vi "Spectrometer iHR320 Control Panel (No Objects).vi"(8 "error in (no error)":errorcluster) -> (0 "error out":errorcluster)   [LabVIEW 2012]
doc: "(Dynamic) A user-level application that simulates the physical front panel of the Instrument. Provide the user with buttons to manually control features of the instrument, and provide indicators of its current state."
panel:
  in  "Set Filter":bool
  out "Filter Index":i32(ring)=1 items=["Filter 1"=1, "Empty"=2, "Empty"=3, "Empty"=4, "Filter 2"=5, "Filter 3"=6]
  in  "Filter Index Set":i32(ring)=1 items=["Filter 1"=1, "Empty"=2, "Empty"=3, "Empty"=4, "Filter 2"=5, "Filter 3"=6]
  in  "Copy actual to set":bool
  in  "Populate fields with member data":bool
  out "Grating":u16(ring)=1 items=["1200"=1, "600"=2]
  in  "Set Grating":bool
  in  "stop":bool
  in  "Read to control":bool
  in  "Read":bool
  in  "Go To Wavelength":bool
  in  "Set Slit":bool
  in  "Grating set":u16(ring)=1 items=["1200"=1, "600"=2]
  out "Wavelength":dbl[unit]
  in  "Wavelength Set":dbl[unit]
  out "Exit Slit":dbl[unit]
  in  "Exit Slit Set":dbl[unit]
  out "Entrance Slit":dbl[unit]
  in  "Entrance  set":dbl[unit]
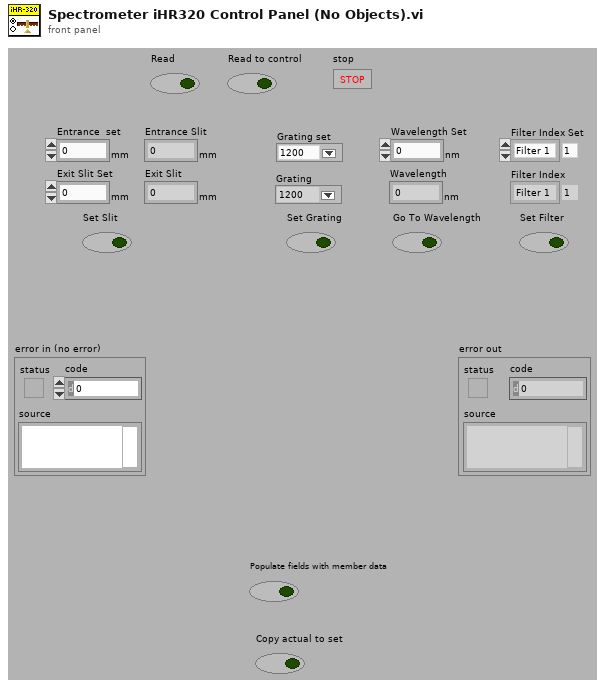
[diagram p1: front panel]
types:
  T1 = cluster{"Wavelength":dbl[unit], "Entrance slit width":dbl[unit], "Exit slit width":dbl[unit], "Init":cluster{"Initialized?":bool, "Emulating?":bool}, "Grating":cluster{"Groove Density":dbl[unit], "Blaze Wavelength":string, "Turrent Position":u16}, "RefNum":refnum<k7>, "Unique ID":string, "FW RefNum":refnum<k7>, "FW Unique ID":string, "Filter Index":i32}
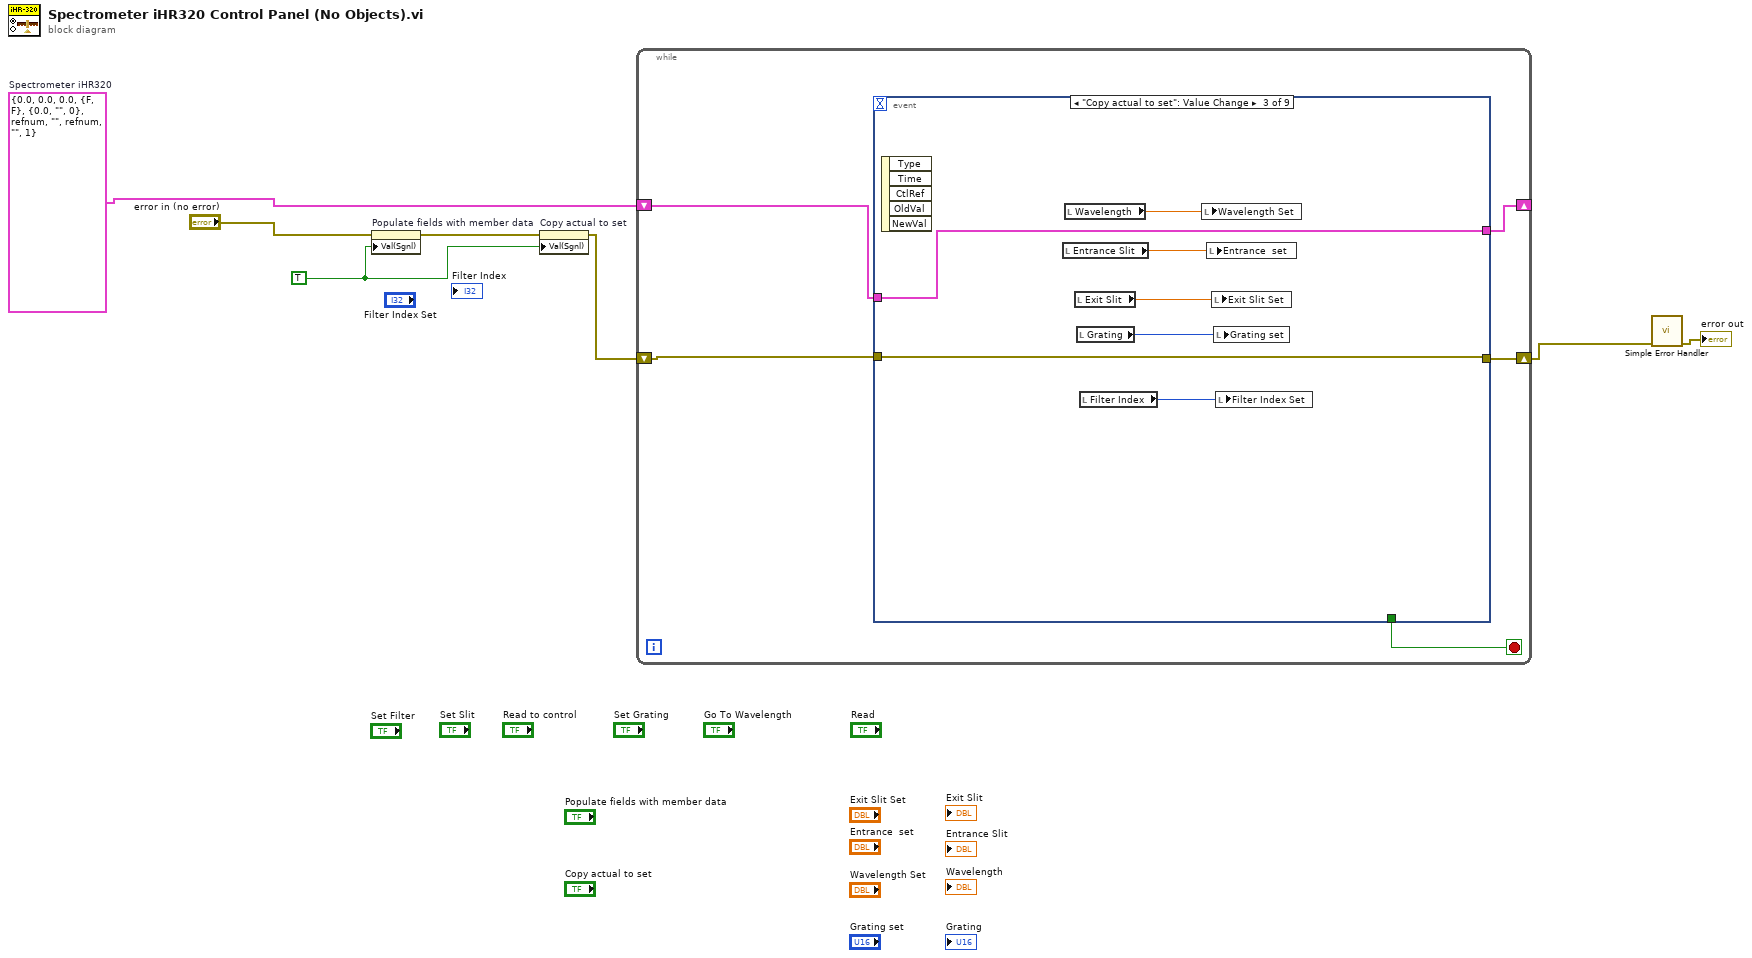
[diagram p0: block diagram]
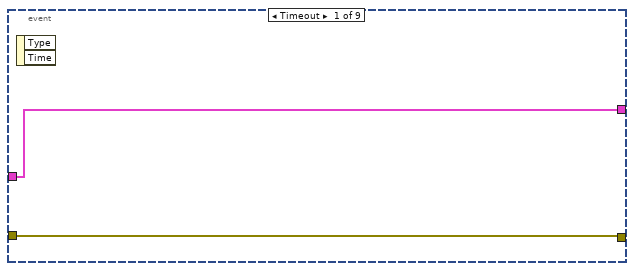
[diagram p2: hidden frame]
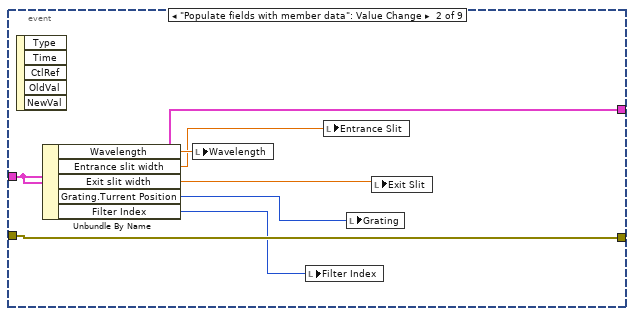
[diagram p3: hidden frame]
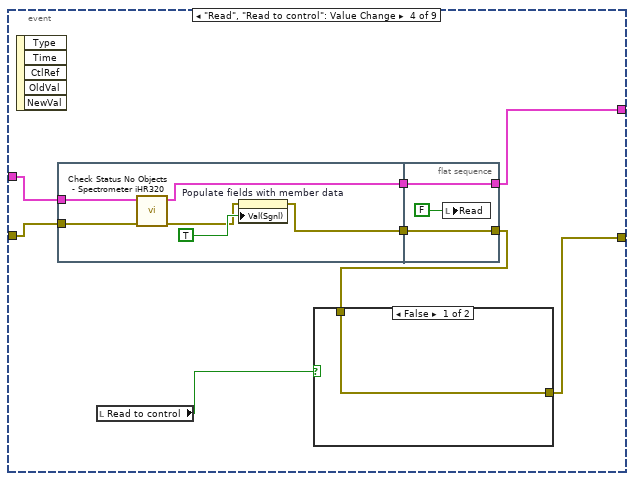
[diagram p4: hidden frame]
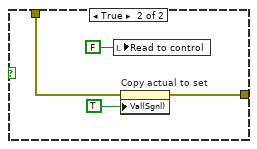
[diagram p5: hidden frame]
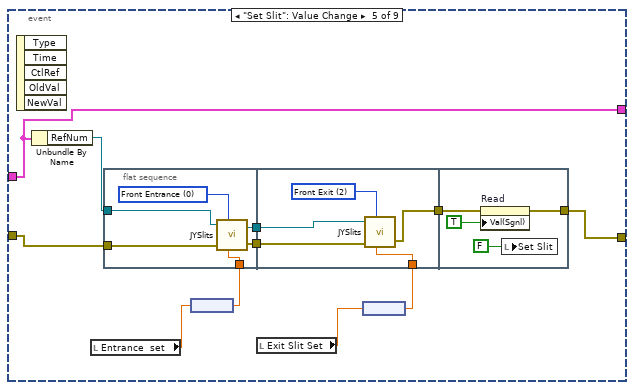
[diagram p6: hidden frame]
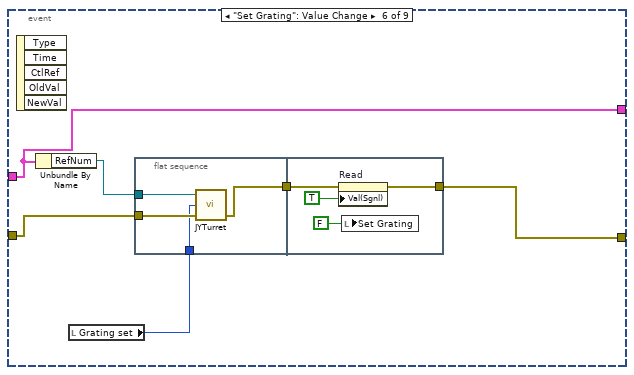
[diagram p7: hidden frame]
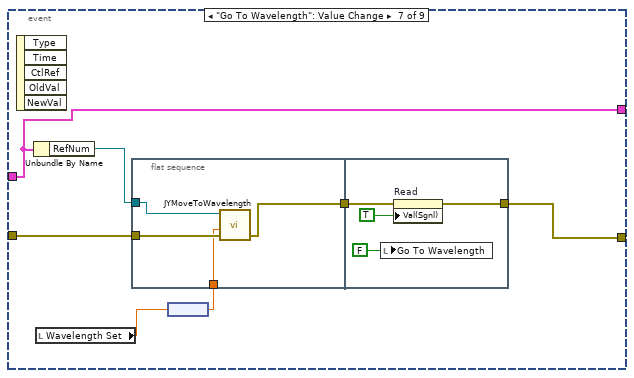
[diagram p8: hidden frame]
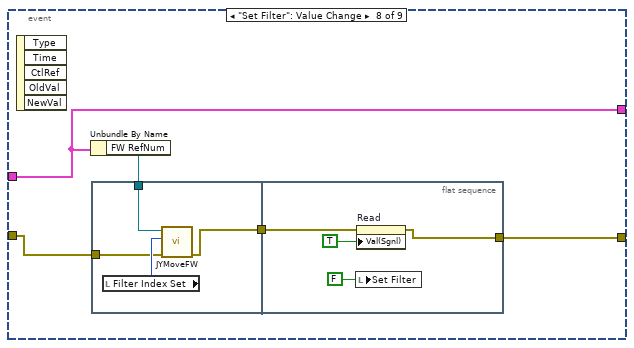
[diagram p9: hidden frame]
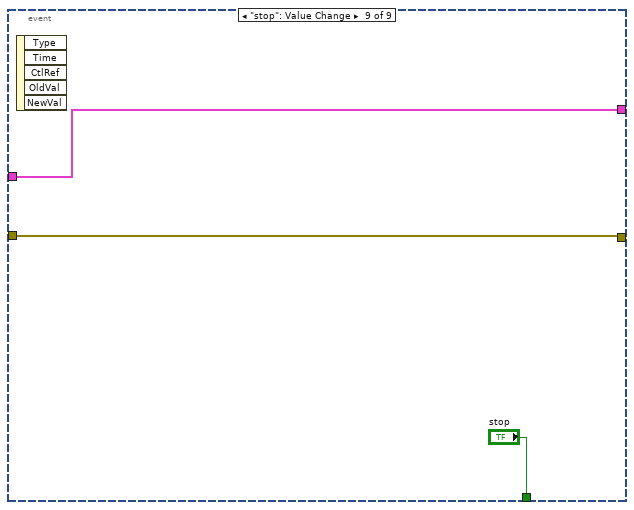
[diagram p10: hidden frame]
diagram:
  w2 = T1 {"Wavelength"=0.0, "Entrance slit width"=0.0, "Exit slit width"=0.0, "Init"={"Initialized?"=FALSE, "Emulating?"=FALSE}, "Grating"={"Groove Density"=0.0, "Blaze Wavelength"="", "Turrent Position"=0}, "RefNum"=refnum, "Unique ID"="", "FW RefNum"=refnum, "FW Unique ID"="", "Filter Index"=1}  # Spectrometer iHR320
  w6 = TRUE ("Value (Signaling)")
  n1 = property on="Populate fields with member data" class="Bool (strict)"(error in="error in (no error)", "Val(Sgnl)"=w6) -> (error out=w7:errorcluster)  [unwired: 1 in, 1 out]
  n2 = property on="Copy actual to set" class="Bool (strict)"(error in=w7, "Val(Sgnl)"=w6) -> (error out=w5:errorcluster)  [unwired: 1 in, 1 out]
  n3 = while {
    shift-right: [w10] -> w1
    shift-left: w5 -> [w12]
    shift-right: [w9] -> _
    shift-left: w2 -> [w11]
    stop <- w8 stop-if-true
    n4 = event shown="[2] \"Copy actual to set\": Value Change" {
      selector: _ -> [_ _ _ _ _ _ _ _ _]
      dyn-events: _ -> [_ _ _ _ _ _ _ _ _]
      timeout: _ -> [_ _ _ _ _ _ _ _ _]
      tunnel: w12 -> [w14 w17 w23 w36 w58 w81 w97 w108 w121]
      tunnel: w11 -> [w13 w16 w24 w35 w51 w77 w91 w110 w120]
      tunnel: [w14 w17 w23 w30 w59 w79 w92 w106 w121] -> w10
      tunnel: [w13 w16 w24 w29 w51 w77 w91 w110 w120] -> w9
      tunnel: [_ _ _ _ _ _ _ _ "stop"] -> w8
      event Timeout {
        n5 = event-data() -> ()  [unwired: 1 in, 2 out]
      }
      event "Populate fields with member data": Value Change {
        n6 = event-data() -> ()  [unwired: 1 in, 5 out]
        n7 = Unbundle By Name(w16) -> ("Wavelength"=w21:dbl[unit], "Entrance slit width"=w20:dbl[unit], "Exit slit width"=w19:dbl[unit], "Grating.Turrent Position"=w18:u16, "Filter Index"=w15:i32)
        n8 = local write "Wavelength"(w21) -> ()
        n9 = local write "Filter Index"(w15) -> ()
        n10 = local write "Entrance Slit"(w20) -> ()
        n11 = local write "Grating"(w18) -> ()
        n12 = local write "Exit Slit"(w19) -> ()
      }
      event "Copy actual to set": Value Change {
        n13 = event-data() -> ()  [unwired: 1 in, 5 out]
        n14 = local read "Entrance Slit"() -> (w27:dbl[unit])
        n15 = local read "Wavelength"() -> (w28:dbl[unit])
        n16 = local read "Exit Slit"() -> (w26:dbl[unit])
        n17 = local read "Grating"() -> (w25:u16)
        n18 = local read "Filter Index"() -> (w22:i32)
        n19 = local write "Wavelength Set"(w28) -> ()
        n20 = local write "Entrance  set"(w27) -> ()
        n21 = local write "Exit Slit Set"(w26) -> ()
        n22 = local write "Grating set"(w25) -> ()
        n23 = local write "Filter Index Set"(w22) -> ()
      }
      event "Read", "Read to control": Value Change {
        n24 = event-data() -> ()  [unwired: 1 in, 5 out]
        n25 = flat-sequence {
          tunnel: w36 -> [w44]
          tunnel: w35 -> [w43]
          tunnel: [w46] -> w34
          tunnel: [w42] -> w33
          tunnel: [w49] -> w31
          tunnel: w34 -> [w49]
          tunnel: [w48] -> w29
          tunnel: w33 -> [w48]
          frame #0 {
            n26 = call "Check Status No Objects - Spectrometer iHR320.vi"("error in (no error)"=w44, "Spectrometer iHR320 in 2"=w43) -> ("error out"=w45:errorcluster, "Spectrometer iHR320 out"=w42:T1)  [unwired: 6 in, 2 out]
            n27 = property on="Populate fields with member data" class="Bool (strict)"(error in=w45, "Val(Sgnl)"=TRUE ("Value (Signaling)")) -> (error out=w46:errorcluster)  [unwired: 1 in, 1 out]
          }
          frame #1 {
            n28 = local write "Read"(FALSE ("Read")) -> ()
          }
        }
        n29 = local read "Read to control"() -> (w32:bool)
        n30 = case shown="False" w32 {
          tunnel: w31 -> [w37 w39]
          tunnel: [w37 w38] -> w30
          frame False {
          }
          frame True {
            n31 = local write "Read to control"(FALSE ("Read to control")) -> ()
            n32 = property on="Copy actual to set" class="Bool (strict)"(error in=w39, "Val(Sgnl)"=TRUE ("Value (Signaling)")) -> (error out=w38:errorcluster)  [unwired: 1 in, 1 out]
          }
        }
      }
      event "Set Slit": Value Change {
        n33 = event-data() -> ()  [unwired: 1 in, 5 out]
        n34 = Unbundle By Name(w51) -> ("RefNum"=w57:refnum<k7>)
        n35 = local read "Entrance  set"() -> (w55:dbl[unit])
        n36 = flat-sequence {
          tunnel: [w66] -> w61
          tunnel: w58 -> [w65]
          tunnel: w57 -> [w64]
          tunnel: [w63] -> w56
          tunnel: w54 -> [w62]
          tunnel: w61 -> [w71]
          tunnel: [w70] -> w60
          tunnel: w56 -> [w69]
          tunnel: w52 -> [w68]
          tunnel: w60 -> [w74]
          tunnel: [w73] -> w59
          frame #0 {
            w67 = u16 0 items=["Front Entrance", "Side Entrance", "Front Exit", "Side Exit", "First Intermediate", "Second Intermediate"] ("Slit")
            n37 = call "JYSlits.vi"("JYMONOLib.IJYMonoReqd In"=w64, "Slit"=w67, "error in (no error)"=w65, "Slit Width"=w62) -> ("JYMONOLib.IJYMonoReqd Out"=w63:refnum<k7>, "error out"=w66:errorcluster)  [unwired: 1 in]
          }
          frame #1 {
            w72 = u16 2 items=["Front Entrance", "Side Entrance", "Front Exit", "Side Exit", "First Intermediate", "Second Intermediate"] ("Slit")
            n38 = call "JYSlits.vi"("JYMONOLib.IJYMonoReqd In"=w69, "Slit"=w72, "error in (no error)"=w71, "Slit Width"=w68) -> ("error out"=w70:errorcluster)  [unwired: 1 in, 1 out]
          }
          frame #2 {
            n39 = property on="Read" class="Bool (strict)"(error in=w74, "Val(Sgnl)"=TRUE ("Value (Signaling)")) -> (error out=w73:errorcluster)  [unwired: 1 in, 1 out]
            n40 = local write "Set Slit"(FALSE ("Set Slit")) -> ()
          }
        }
        n41 = node(w55) -> (w54:dbl)
        n42 = local read "Exit Slit Set"() -> (w53:dbl[unit])
        n43 = node(w53) -> (w52:dbl)
      }
      event "Set Grating": Value Change {
        n44 = event-data() -> ()  [unwired: 1 in, 5 out]
        n45 = Unbundle By Name(w77) -> ("RefNum"=w82:refnum<k7>)
        n46 = local read "Grating set"() -> (w78:u16)
        n47 = flat-sequence {
          tunnel: w82 -> [w86]
          tunnel: w81 -> [w85]
          tunnel: [w84] -> w80
          tunnel: w78 -> [w83]
          tunnel: w80 -> [w88]
          tunnel: [w87] -> w79
          frame #0 {
            n48 = call "JYTurret.vi"("error in (no error)"=w85, "Grating Index"=w83, "JYMONOLib.IJYMonoReqd In"=w86) -> ("error out"=w84:errorcluster)  [unwired: 2 out]
          }
          frame #1 {
            n49 = property on="Read" class="Bool (strict)"(error in=w88, "Val(Sgnl)"=TRUE ("Value (Signaling)")) -> (error out=w87:errorcluster)  [unwired: 1 in, 1 out]
            n50 = local write "Set Grating"(FALSE ("Set Grating")) -> ()
          }
        }
      }
      event "Go To Wavelength": Value Change {
        n51 = event-data() -> ()  [unwired: 1 in, 5 out]
        n52 = Unbundle By Name(w91) -> ("RefNum"=w95:refnum<k7>)
        n53 = local read "Wavelength Set"() -> (w94:dbl[unit])
        n54 = flat-sequence {
          tunnel: w97 -> [w101]
          tunnel: [w100] -> w96
          tunnel: w95 -> [w99]
          tunnel: w93 -> [w98]
          tunnel: w96 -> [w103]
          tunnel: [w102] -> w92
          frame #0 {
            n55 = call "JYMoveToWavelength.vi"("error in (no error)"=w101, "Target WL"=w98, "RefNum In"=w99) -> ("error out"=w100:errorcluster)  [unwired: 1 in, 2 out]
          }
          frame #1 {
            n56 = local write "Go To Wavelength"(FALSE ("Go To Wavelength")) -> ()
            n57 = property on="Read" class="Bool (strict)"(error in=w103, "Val(Sgnl)"=TRUE ("Value (Signaling)")) -> (error out=w102:errorcluster)  [unwired: 1 in, 1 out]
          }
        }
        n58 = node(w94) -> (w93:dbl)
      }
      event "Set Filter": Value Change {
        n59 = event-data() -> ()  [unwired: 1 in, 5 out]
        n60 = Unbundle By Name(w110) -> ("FW RefNum"=w109:refnum<k7>)
        n61 = flat-sequence {
          tunnel: w109 -> [w114]
          tunnel: w108 -> [w112]
          tunnel: [w111] -> w107
          tunnel: w107 -> [w116]
          tunnel: [w115] -> w106
          frame #0 {
            n62 = local read "Filter Index Set"() -> (w113:i32)
            n63 = call "JYMoveFW.vi"("error in (no error)"=w112, "Filter Index"=w113, "FW RefNum In"=w114) -> ("error out"=w111:errorcluster)  [unwired: 7 in, 1 out]
          }
          frame #1 {
            n64 = local write "Set Filter"(FALSE ("Set Filter")) -> ()
            n65 = property on="Read" class="Bool (strict)"(error in=w116, "Val(Sgnl)"=TRUE ("Value (Signaling)")) -> (error out=w115:errorcluster)  [unwired: 1 in, 1 out]
          }
        }
      }
      event "stop": Value Change {
        n66 = event-data() -> ()  [unwired: 1 in, 5 out]
      }
    }
  }
  n67 = call <vilib>:"Simple Error Handler.vi"("error in (no error)"=w1) -> ("error out"=→"error out":errorcluster)  [unwired: 4 in, 4 out]
